vi "MonitorActiveProject.vi"(10 "Active Project Changed":refnum<user-event>) -> ()   [LabVIEW 2017, in "TestExplorer.lvlib"]
doc: "Generates a user event when the active project in the current application instance changed. This VI keeps running until the specified user event is destroyed."
uses:
  TestExplorer.lvlib
  b8ae5672-8134-400f-a408-93b2af799a79.vi
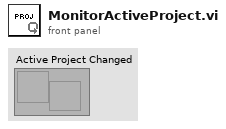
[diagram p1: front panel]
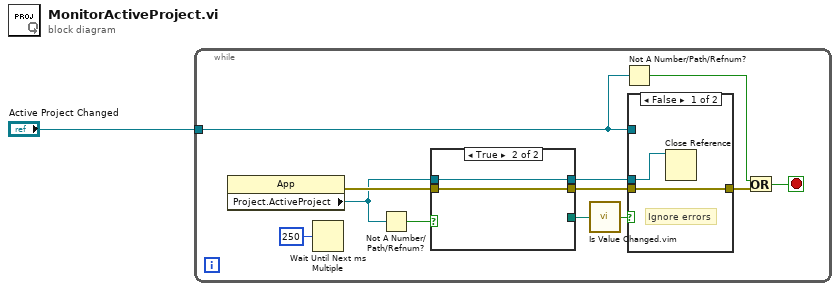
[diagram p0: block diagram]
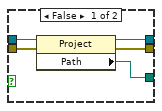
[diagram p2: hidden frame]
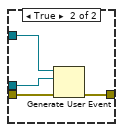
[diagram p3: hidden frame]
diagram:
  n1 = while {
    tunnel: "Active Project Changed" -> [w3]
    stop <- w4 stop-if-true
    n2 = property class="App"() -> (error out=w13:errorcluster, "Project.ActiveProject"=w7:refnum<vi>)  [unwired: 2 in, 1 out]
    n3 = Wait Until Next ms Multiple(millisecond multiple=u32 250) -> ()  [unwired: 1 out]
    n4 = Not A Number/Path/Refnum?(number/path/refnum=w7) -> (NaN/Path/Refnum?=w6:bool)
    n5 = case shown="True" w6 {
      tunnel: w13 -> [w18 w19]
      tunnel: w7 -> [w17 w20]
      tunnel: [w16 _] -> w12
      tunnel: [w15 w20] -> w10
      tunnel: [w14 w19] -> w9
      frame False {
        n6 = property class="Project"(reference=w17, error in=w18) -> (reference out=w15:refnum<vi>, error out=w14:errorcluster, "Path"=w16:path)
      }
      frame True {
      }
    }
    n7 = call "Is Value Changed.vim"("value"=w12) -> ("changed or first call?"=w11:bool)
    n8 = Not A Number/Path/Refnum?(number/path/refnum=w3) -> (NaN/Path/Refnum?=w2:bool)
    n9 = case shown="False" w11 {
      tunnel: w3 -> [_ w26]
      tunnel: w10 -> [w22 w25]
      tunnel: w9 -> [w21 w24]
      tunnel: [w21 w23] -> w5
      frame False {
        # "Ignore errors"
        n10 = Close Reference(reference=w22) -> ()  [unwired: 1 in, 1 out]
      }
      frame True {
        n11 = Generate User Event(user event=w26, event data cluster=w25, error in=w24) -> (error out=w23:errorcluster)  [unwired: 1 in, 1 out]
      }
    }
    n12 = Or(x=w2, y=w5) -> (x .or. y?=w4:bool)
  }
